vi "Start Listener SMO--delete.vi"(8 "error in (no error)":errorcluster, 11 "RemoteControl in":refnum<class "RemoteControl.lvclass">) -> (0 "error out":errorcluster, 3 "RemoteControl out":refnum<class "RemoteControl.lvclass">)   [LabVIEW 2019]
uses:
  RemoteControl.lvclass
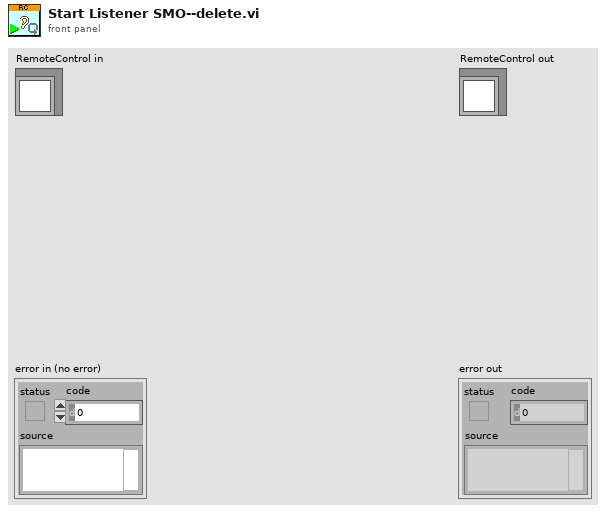
[diagram p1: front panel]
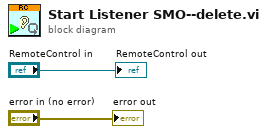
[diagram p0: block diagram]
diagram:
  "error out" <- "error in (no error)"
  "RemoteControl out" <- "RemoteControl in"
